vi "Calculate Wavelength.vi"(8 "error in (no error)":errorcluster, 10 "Number of Pixels (3648)":i32=3648, 11 "VISA resource name":refnum<visa-resource-name>) -> (0 "error out":errorcluster, 2 "Wavelength (nm)":dbl[](array[numeric]), 3 "VISA resource name out":refnum<visa-resource-name>)   [LabVIEW 2023, in "Ocean Optics 2000 4000.lvlib"]
doc: "Calculate the wavelength from each pixel number."
uses:
  <instrlib>/Ocean Optics 2000 4000/Ocean Optics 2000 4000.lvlib
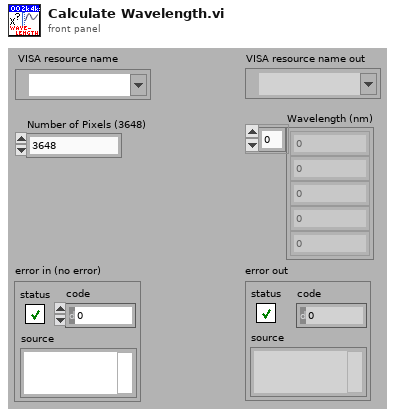
[diagram p1: front panel]
types:
  T1 = cluster{"Start Pixel":i32, "Stop Pixel":i32, "Start Black":i32[], "Stop Black":i32[]}
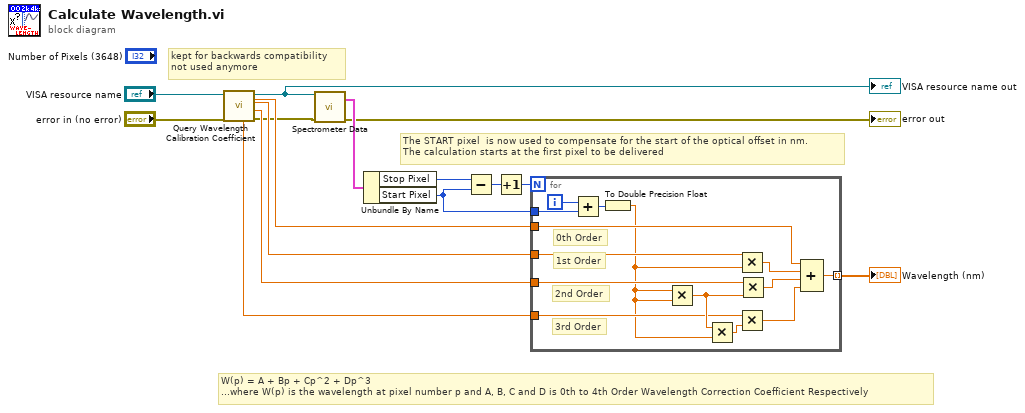
[diagram p0: block diagram]
diagram:
  # "The START pixel  is now used to compensate for the start of the optical offset in nm.\nThe calculation starts at the first pixel to be delivered"
  # "kept for backwards compatibility\nnot used anymore"
  # "W(p) = A + Bp + Cp^2 + Dp^3  \n...where W(p) is the wavelength at pixel number p and A, B, C and D is 0th to 4th Order Wavelength Correction Coefficient Respectively"
  n1 = call <instrlib>:"Query Wavelength Calibration Coefficient.vi"("error in (no error)"="error in (no error)", "VISA resource name"="VISA resource name") -> ("error out"=w6:errorcluster, "2nd Order Wavelength Calibration Coefficient"=w13:dbl, "1st Order Wavelength Calibration Coefficient"=w14:dbl, "VISA resource name out"=w5:refnum<visa-resource-name>, "3rd Order Wavelength Calibration Coefficient"=w12:dbl, "0th Order Wavelength Calibration Coefficient"=w15:dbl)  [unwired: 4 out]
  "VISA resource name out" <- w5
  n2 = call <instrlib>:"Spectrometer Data.vi"("VISA resource name"=w5, "error in (no error)"=w6) -> ("Pixels"=w9:T1, "error out"=→"error out":errorcluster)  [unwired: 8 in, 4 out]
  n3 = Unbundle By Name(w9) -> ("Stop Pixel"=w3:i32, "Start Pixel"=w1:i32)
  n4 = Subtract(x=w3, y=w1) -> (x-y=w10:i32)
  n5 = Increment(x=w10) -> (x+1=w2:i32)
  n6 = for {
    N: w2 -> [_]
    tunnel: w14 -> [w29]
    tunnel: w15 -> [w25]
    tunnel: w12 -> [w23]
    tunnel: [w21] -> w11 mode=indexing
    tunnel: w13 -> [w20]
    tunnel: w1 -> [w16]
    i -> [w17]
    # "3rd Order"
    # "2nd Order"
    # "1st Order"
    # "0th Order"
    n7 = Add(x=w17, y=w16) -> (x+y=w19:i32)
    n8 = To Double Precision Float(number=w19) -> (double precision float=w18:dbl)
    n9 = Multiply(x=w18, y=w18) -> (x*y=w26:dbl)
    n10 = Multiply(x=w26, y=w18) -> (x*y=w24:dbl)
    n11 = Multiply(x=w29, y=w18) -> (x*y=w27:dbl)
    n12 = Multiply(x=w23, y=w24) -> (x*y=w22:dbl)
    n13 = Multiply(x=w20, y=w26) -> (x*y=w28:dbl)
    n14 = Compound Arithmetic op=ADD(w25, w27, w28, w22) -> (w21:dbl)
  }
  "Wavelength (nm)" <- w11
